vi "test_spline_nak.vi"() -> ()   [LabVIEW 2009]
doc: "Copyright (C) 2009, Stepan A. Baranov\nweb: http://www.OCTLab.org/\nemail: stepan@baranov.su"
uses:
  <vilib>/Analysis/NI_AALPro.lvlib
  OCTLib.dll
panel:
  out "error out":errorcluster
  in  "Small/Big":bool
  out "XY Graph":cluster{"Y":dbl[], "Y":dbl[]}[](graph)
  out "Waveform Graph":dbl[][](graph)
  out "width":i32
  out "height":i32
  out "loop #":i32
  out "RSM_STAT time":u32
  out "LabView time":u32
  out "RSM_STAT Array":dbl[][](array[numeric])
  out "LabView Array":dbl[][](array[numeric])
  in  "stop":bool
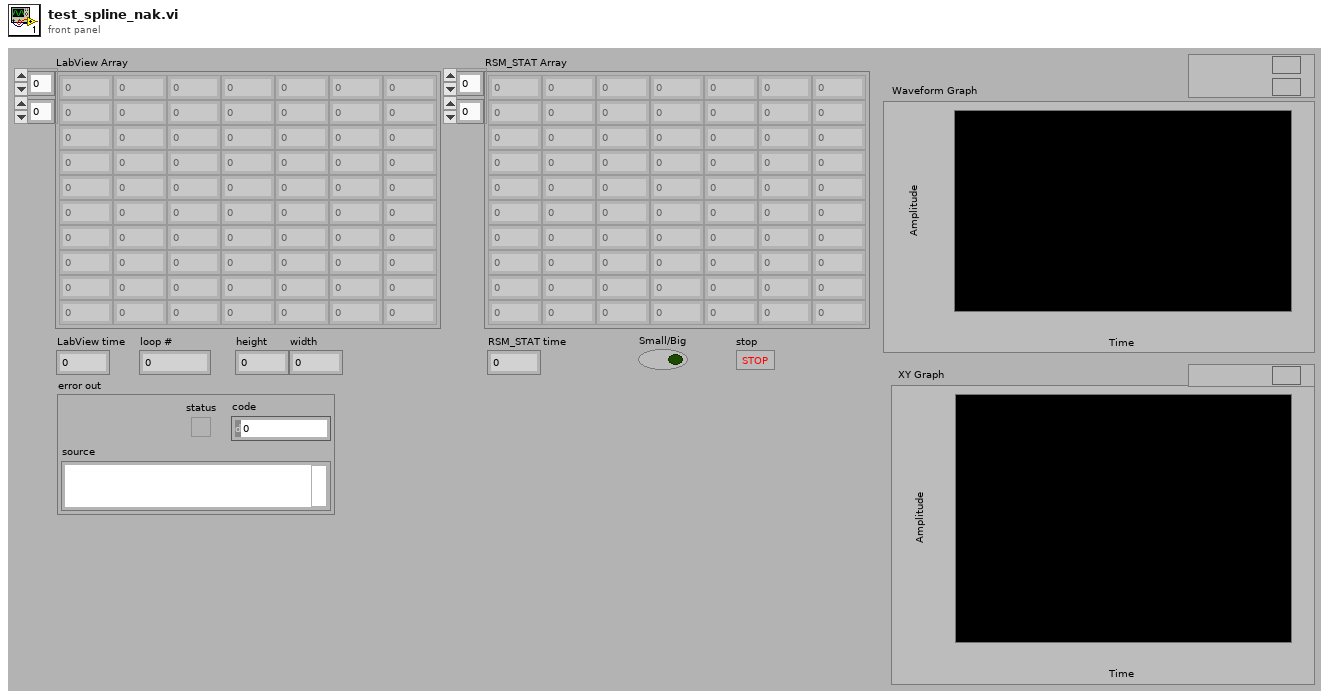
[diagram p1: front panel]
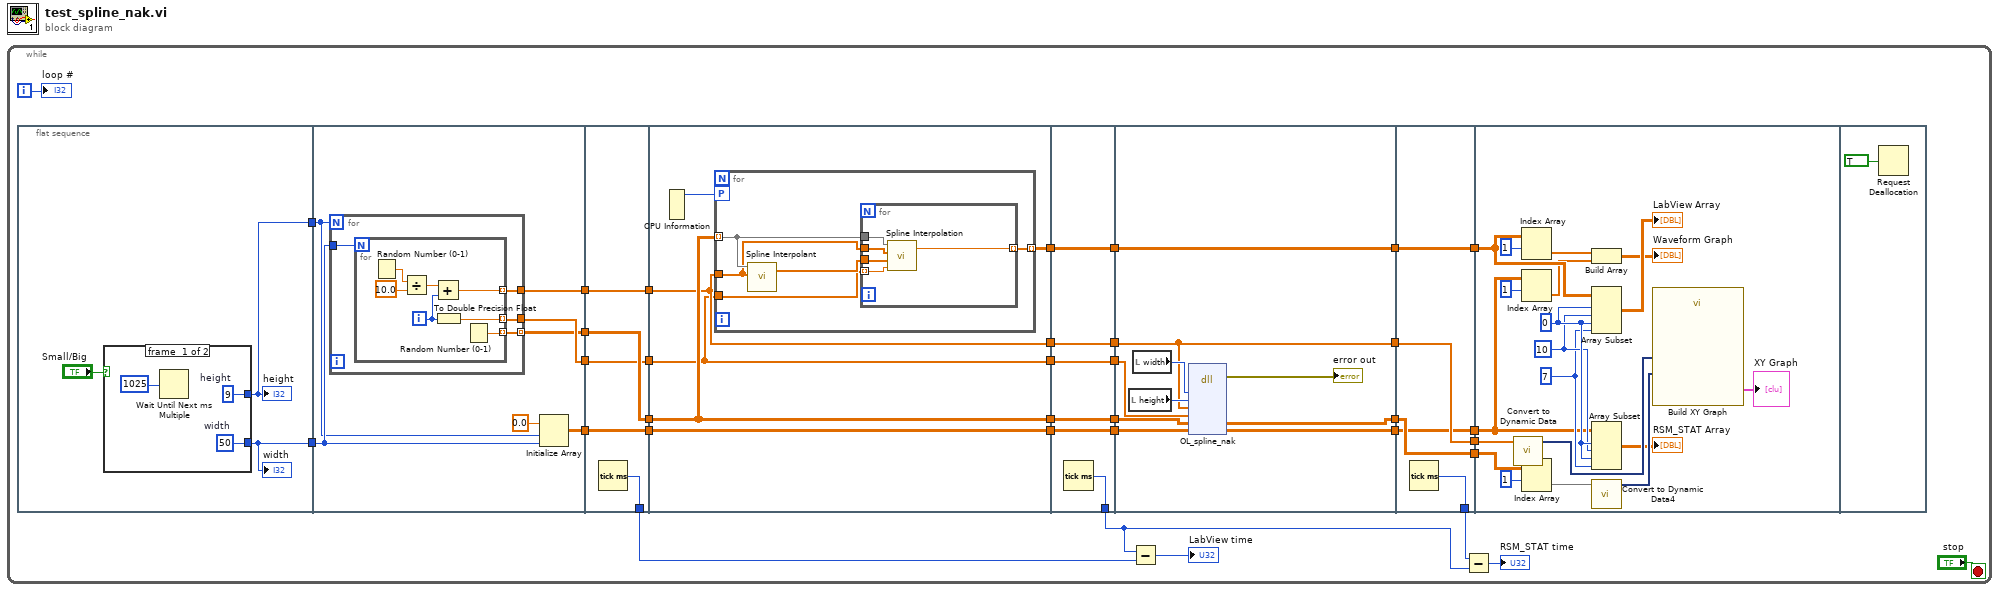
[diagram p0: block diagram]
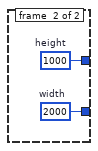
[diagram p2: hidden frame]
diagram:
  n1 = while {
    i -> [w29]
    stop <- "stop" stop-if-true
    n2 = flat-sequence {
      tunnel: [w37] -> w26
      tunnel: [w38] -> w25
      tunnel: [w46] -> w27
      tunnel: w26 -> [w45]
      tunnel: w25 -> [w44]
      tunnel: [w47] -> w24
      tunnel: [w49] -> w21
      tunnel: [w48] -> w14
      tunnel: [w66] -> w34
      tunnel: [w65] -> w28
      tunnel: w27 -> [w65]
      tunnel: w24 -> [w64]
      tunnel: [w64] -> w23
      tunnel: [w63] -> w22
      tunnel: w21 -> [w63]
      tunnel: w14 -> [w62]
      tunnel: [w62] -> w13
      tunnel: w28 -> [w70]
      tunnel: w23 -> [w71]
      tunnel: w22 -> [w69]
      tunnel: [w71] -> w19
      tunnel: [w70] -> w17
      tunnel: [w69] -> w15
      tunnel: w13 -> [w68]
      tunnel: [w68] -> w12
      tunnel: [w67] -> w1
      tunnel: [w88] -> w31
      tunnel: [w87] -> w20
      tunnel: w19 -> [w87]
      tunnel: [w86] -> w18
      tunnel: w17 -> [w86]
      tunnel: [w85] -> w16
      tunnel: w15 -> [w85]
      tunnel: w12 -> [w84]
      tunnel: [w84] -> w11
      tunnel: [w83] -> w2
      tunnel: w1 -> [w83]
      tunnel: w20 -> [w93]
      tunnel: w18 -> [w92]
      tunnel: w16 -> [w96]
      tunnel: w11 -> [w95]
      tunnel: [w89] -> w9
      tunnel: [w92] -> w7
      tunnel: [w91] -> w5
      tunnel: [w90] -> w3
      tunnel: w2 -> [w90]
      tunnel: [w103] -> w32
      tunnel: [w102] -> w10
      tunnel: w9 -> [w102]
      tunnel: [w101] -> w8
      tunnel: w7 -> [w101]
      tunnel: [w100] -> w6
      tunnel: w5 -> [w100]
      tunnel: [w99] -> w4
      tunnel: w3 -> [w99]
      tunnel: w10 -> [w110]
      tunnel: w8 -> [w109]
      tunnel: w6 -> [w108]
      tunnel: w4 -> [w107]
      frame #0 {
        n3 = case shown="False" "Small/Big" {
          tunnel: [w41 w42] -> w38
          tunnel: [w40 w43] -> w37
          frame #0 {
            w40 = 50  # width
            w41 = 9  # height
            n4 = Wait Until Next ms Multiple(millisecond multiple=u32 1025) -> ()  [unwired: 1 out]
          }
          frame #1 {
            w43 = 2000  # width
            w42 = 1000  # height
          }
        }
        "height" <- w38
        "width" <- w37
      }
      frame #1 {
        n5 = for {
          N: w44 -> [_]
          tunnel: w45 -> [w54]
          tunnel: [w53] -> w46
          tunnel: [w52] -> w47 mode=indexing
          tunnel: [w51] -> w49
          n6 = for {
            N: w54 -> [_]
            tunnel: [w57] -> w53 mode=indexing
            tunnel: [w61] -> w52 mode=indexing
            tunnel: [w55] -> w51 mode=indexing
            i -> [w56]
            n7 = Random Number (0-1)() -> (number: 0 to 1=w60:dbl)
            n8 = Divide(x=w60, y=10.0) -> (x/y=w59:dbl)
            n9 = Add(x=w59, y=w56) -> (x+y=w57:dbl)
            n10 = To Double Precision Float(number=w56) -> (double precision float=w55:dbl)
            n11 = Random Number (0-1)() -> (number: 0 to 1=w61:dbl)
          }
        }
        n12 = Initialize Array(0.0 ("element"), w44, w45) -> (w48:dbl[][])
      }
      frame #2 {
        n13 = Tick Count (ms)() -> (millisecond timer value=w66:u32)
      }
      frame #3 {
        n14 = CPU Information() -> (4:w72:i32)  [unwired: 3 out]
        n15 = for {
          tunnel: w70 -> [w75]
          workers-P: w72 -> [_]
          tunnel: w71 -> [w76] mode=indexing
          tunnel: w69 -> [w74]
          tunnel: [w73] -> w67 mode=indexing
          n16 = call <vilib>:"Spline Interpolant.vi"("X"=w75, "Y"=w76) -> ("Interpolant"=w77:dbl[])  [unwired: 2 in, 1 out]
          n17 = for {
            tunnel: w77 -> [w82]
            tunnel: w76 -> [w81]
            tunnel: w75 -> [w80]
            tunnel: w74 -> [w79] mode=indexing
            tunnel: [w78] -> w73 mode=indexing
            n18 = call <vilib>:"Spline Interpolation.vi"("x value"=w79, "Interpolant"=w82, "X"=w80, "Y"=w81) -> ("interpolation value"=w78:dbl)  [unwired: 1 out]
          }
        }
      }
      frame #4 {
        n19 = Tick Count (ms)() -> (millisecond timer value=w88:u32)
      }
      frame #5 {
        n20 = local read "height"() -> (w97:i32)
        n21 = local read "width"() -> (w98:i32)
        n22 = dll-call lib="OCTLib.dll" fn="OL_spline_nak"("width"=w98, "height"=w97, "X"=w92, "XX"=w96, "in"=w93, "out"=w95) -> (error out=→"error out":errorcluster, "in"=w89:dbl[][], "out"=w91:dbl[][])  [unwired: 8 in, 1 out]
      }
      frame #6 {
        n23 = Tick Count (ms)() -> (millisecond timer value=w103:u32)
      }
      frame #7 {
        w121 = 10 ("length")
        w120 = 7 ("length")
        w122 = 0 ("index")
        n24 = call "Convert to Dynamic Data"("Array"=w109) -> ("Dynamic Data Type"=w112:dynamicdata)  [unwired: 3 in]
        n25 = Index Array(array=w107, index (row)=1) -> (element=w106:dbl[])  [unwired: 1 in]
        n26 = Index Array(array=w108, index (row)=1) -> (element=w105:dbl[])  [unwired: 1 in]
        n27 = Index Array(array=w110, index (row)=1) -> (element=w114:dbl[])  [unwired: 1 in]
        n28 = Build Array(w106, w105) -> (→"Waveform Graph":dbl[][])
        n29 = Array Subset(array=w107, index (row)=w122, length (row)=w121, index (col)=w122, length (col)=w120) -> (→"LabView Array":dbl[][])
        n30 = Array Subset(array=w108, index (row)=w122, length (row)=w121, index (col)=w122, length (col)=w120) -> (→"RSM_STAT Array":dbl[][])
        n31 = call "Convert to Dynamic Data4"("Array"=w114) -> ("Dynamic Data Type"=w113:dynamicdata)  [unwired: 3 in]
        n32 = call "Build XY Graph"("Y Input"=w113, "X Input"=w112) -> ("XY Graph"=→"XY Graph":cluster{"Y":dbl[], "Y":dbl[]}[])  [unwired: 8 in, 1 out]
      }
      frame #8 {
        n33 = Request Deallocation(TRUE ("flag")) -> ()
      }
    }
    n34 = Subtract(x=w31, y=w34) -> (x-y=→"LabView time":u32)
    n35 = Subtract(x=w32, y=w31) -> (x-y=→"RSM_STAT time":u32)
    "loop #" <- w29
  }
